vi "StatusUpdateByModID.vi"(8 "error in (no error)":errorcluster, 10 "Status":string, 11 "Accessors:Module ID":i32) -> (0 "error out":errorcluster)   [LabVIEW 2018, in "AcPwrPlugins.lvlib"]
uses:
  AcPwrPlugins.lvlib
  AcPwrShared/clEventType.ctl
  AcPwrShared/AcPwrShared.lvlib
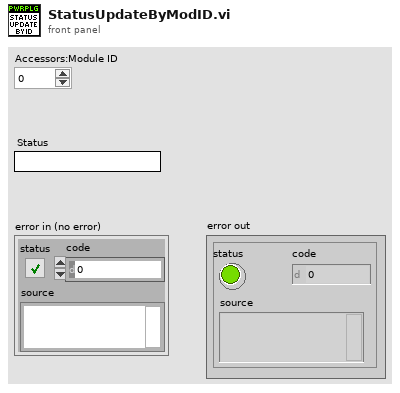
[diagram p1: front panel]
types:
  T1 = typedef "AcPwrShared.lvlib/clEventType.ctl" = cluster{"ModuleID":i32, "Data":variant}
  T2 = typedef "AcPwrShared.lvlib/AcPwrBroadcastEvents.ctl" = cluster{"DidInit":refnum<user-event>, "StatusUpdate":refnum<user-event>, "ErrorReport":refnum<user-event>, "DidStop":refnum<user-event>, "PathToINI":refnum<user-event>, "Measurements":refnum<user-event>, "LoadConfigFile":refnum<user-event>, "GetSettings":refnum<user-event>, "SetSettings":refnum<user-event>, "GetType&ID":refnum<user-event>, "GotSettings":refnum<user-event>, "GotSettingsLV":refnum<user-event>}
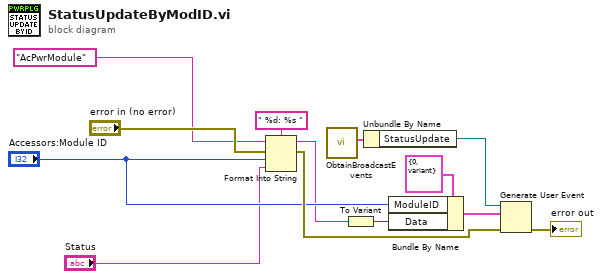
[diagram p0: block diagram]
diagram:
  n1 = Format Into String(format string=" %d: %s ", initial string="AcPwrModule" ("Accessors:ModuleName"), error in="error in (no error)", "Accessors:Module ID", "Status") -> (resulting string=w10:string, error out=w13:errorcluster)
  n2 = call "ObtainBroadcastEvents.vi"() -> ("AcPwrEvents"=w1:T2)  [unwired: 10 in, 1 out]
  n3 = To Variant(anything=w10) -> (Variant=w4:variant)
  n4 = Unbundle By Name(w1) -> ("StatusUpdate"=w2:refnum<user-event>)
  n5 = Bundle By Name(cluster=T1 {"ModuleID"=0, "Data"=variant} ("clBroadcast"), "ModuleID"="Accessors:Module ID", "Data"=w4) -> (w5:T1)
  n6 = Generate User Event(user event=w2, event data cluster=w5, error in=w13) -> (error out=→"error out":errorcluster)  [unwired: 1 in, 1 out]
